vi "Lid Lock Control.vi"(0 "GEA2 Reference In":refnum<k24>, 5 "Action":enum16{"Lock", "Unlock"}(ring), 11 "Error In":errorcluster) -> (4 "GEA2 Reference Out":refnum<k24>, 6 "Pass/Fail?":bool, 8 "Report Text":string, 15 "Error Out":errorcluster)   [LabVIEW 2016, in "2015 VA Washer.lvlib"]
doc: "Use this VI to lock or unlock the lid."
uses:
  Projects/2015 VA Washer.lvlib
  C:/Automation/DLLs/PC Dot Net/GeaCommunication.dll
  Common/LabVIEW GEA2 Toolkit/LabVIEW_GEA2_Toolkit.lvlibp/type defs/Source_Destination.ctl
  Common/LabVIEW GEA2 Toolkit/LabVIEW_GEA2_Toolkit.lvlibp/type defs/ERD Read Data In.ctl
  Common/LabVIEW GEA2 Toolkit/LabVIEW_GEA2_Toolkit.lvlibp/type defs/Data Type.ctl
  Common/LabVIEW GEA2 Toolkit/LabVIEW_GEA2_Toolkit.lvlibp/type defs/ERD Write Data In.ctl
  Common/LabVIEW GEA2 Toolkit/LabVIEW_GEA2_Toolkit.lvlibp
panel:
  in  "Standalone?":bool
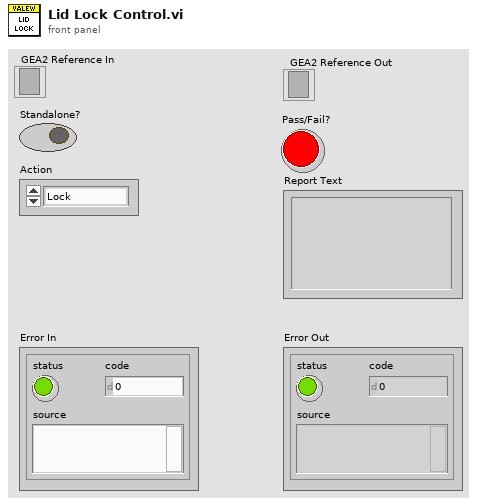
[diagram p1: front panel]
types:
  T1 = enum16{"EQ (==)", "NE (!=)", "GT (>)", "LT (<)", "GE (>=)", "LE (<=)", "GTLT(> <)", "GELE (>= <=)", "GELT (>= <)", "GTLE (> <=)", "LTGT (< >)", "LEGE (<= >=)", "LEGT (<= >)", "LTGE (< >=)", "No Comparison"}
  T2 = typedef "LabVIEW_GEA2_Toolkit.lvlibp/ERD Read Data In.ctl" = cluster{"ERD Number":u16, "Data Type":T3}
  T3 = typedef "LabVIEW_GEA2_Toolkit.lvlibp/Data Type.ctl" = enum16{"string", "boolean", "uint8_t", "uint16_t", "uint32_t", "uint64_t", "int8_t", "int16_t", "int32_t", "int64_t"}
  T4 = typedef "LabVIEW_GEA2_Toolkit.lvlibp/Source_Destination.ctl" = cluster{"Source":u8, "Destination":u8}
  T5 = typedef "LabVIEW_GEA2_Toolkit.lvlibp/ERD Write Data In.ctl" = cluster{"ERD Number":u16, "Data Type":T3, "Data":string}
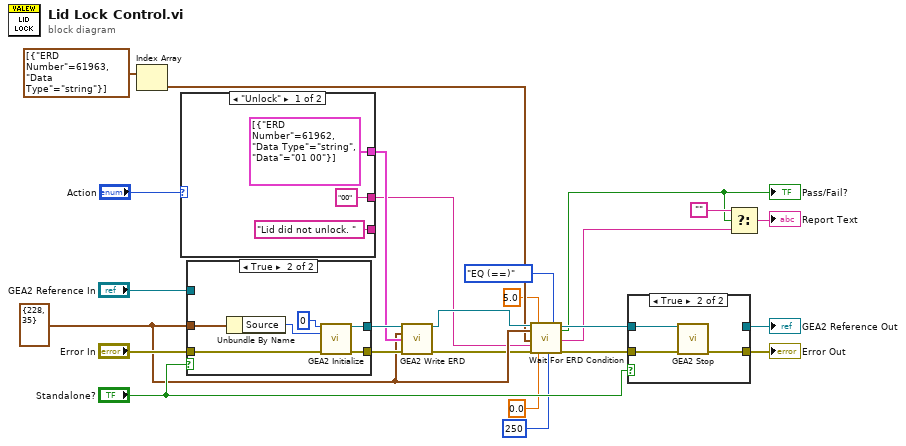
[diagram p0: block diagram]
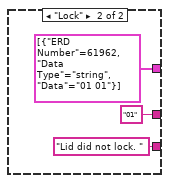
[diagram p2: hidden frame]
diagram:
  w16 = T4 {"Source"=228, "Destination"=35} ("GEA Inputs")
  n1 = Index Array(array=T2[] [{"ERD Number"=61963, "Data Type"=enum."string"}] ("Read ERD List")) -> (element=w8:T2)  [unwired: 1 in]
  n2 = case shown="\"Unlock\"" "Action" {
    tunnel: [T5[] [{"ERD Number"=61962, "Data Type"=enum."string", "Data"="01 00"}] ("Write ERD List") T5[] [{"ERD Number"=61962, "Data Type"=enum."string", "Data"="01 01"}] ("Write ERD List")] -> w18
    tunnel: ["00" ("y") "01" ("y")] -> w7
    tunnel: ["Lid did not unlock. " ("f") "Lid did not lock. " ("f")] -> _
    frame "Unlock" {
    }
    frame "Lock" {
    }
  }
  n3 = case shown="True" "Standalone?" {
    tunnel: "Error In" -> [w32 w39]
    tunnel: [w32 w38] -> w19
    tunnel: "GEA2 Reference In" -> [w33 _]
    tunnel: [w33 w37] -> w25
    tunnel: w16 -> [_ w35]
    frame False {
    }
    frame True {
      n4 = Unbundle By Name(w35) -> ("Source"=w36:u8)
      n5 = call "GEA2 Initialize.vi"("Board Index"=0, "Source Address"=w36, "error in"=w39) -> ("GEA2 Reference Out"=w37:refnum<k24>, "error out"=w38:errorcluster)  [unwired: 10 in, 1 out]
    }
  }
  n6 = call "GEA2 Write ERD.vi"("GEA2 Reference In"=w25, "GEA Inputs"=w16, "Write ERD List"=w18, "Error In"=w19) -> ("GEA2 Reference Out"=w17:refnum<k24>, "Error Out"=w10:errorcluster)  [unwired: 9 in, 1 out]
  n7 = call "Wait For ERD Condition.vi"("GEA2 Reference In"=w17, "GEA Inputs"=w16, "ERD Read Data"=w8, "Expected Low"=w7, "Error In"=w10, "Timeout (s)"=5.0, "Min Exec Time (s)"=0.0, "Loop Rate (ms)"=u32 250, "Comparison"=T1."EQ (==)") -> ("GEA2 Reference Out"=w15:refnum<k24>, "Pass/Fail?"=w6:bool, "Report Text"=w5:string, "Error Out"=w14:errorcluster)  [unwired: 6 in, 1 out]
  "Pass/Fail?" <- w6
  n8 = case shown="True" "Standalone?" {
    tunnel: w14 -> [w41 w44]
    tunnel: [w41 w43] -> w24
    tunnel: [w40 _] -> w23
    tunnel: w15 -> [w40 w42]
    frame False {
    }
    frame True {
      n9 = call "GEA2 Stop.vi"("GEA2 Reference In"=w42, "Error In"=w44) -> ("Error Out"=w43:errorcluster)  [unwired: 13 in]
    }
  }
  "Error Out" <- w24
  "GEA2 Reference Out" <- w23
  n10 = Select(t="", s=w6, f=w5) -> (s? t:f=→"Report Text":string)
